vi "clipattconfiguration.vi"(0 "input cluster":T1, 1 "Channels values 2":i32[](array[numeric]), 2 "vclip":i32[](array[numeric]), 5 "Channels init":i32[](array[numeric])=[2000], 7 "Boolean":bool, 11 "error out 2":errorcluster) -> (6 "vatt":i32[](array[numeric]), 8 "vclip":i32[](array[numeric]), 10 "appended array":i64[](array[numeric]), 15 "error out":errorcluster)   [LabVIEW 2009]
uses:
  <vilib>/Utility/NIReport.llb/NI_report.lvclass
panel:
  in  "Array":dbl[](array[numeric])=[0.05, 0.1, 0.2, 0.3, 0.4, 0.5, 0.6, 0.7, 0.8, 0.9, 1.0, 1.2, 1.4, 1.6, 1.8, 2.0, 2.2, 2.5]
  in  "conf value":i32=100
  out "XY Graph":cluster{"Y":dbl[], "Y":dbl[]}[](graph)
  in  "L1 min invented 2":i32[](array[numeric])=[242, 504, 1031, 2128, 3263, 4418, 5634, 6888]
  in  "L1  50% invented 2":dbl[][](array[numeric])
  in  "L1  50% invented":dbl[][](array[numeric])
  in  "L1 min invented":i32[](array[numeric])=[242, 504, 1031, 2128, 3263, 4418, 5634, 6888]
  out "L1  50%":dbl[][](array[numeric])=[[182.05332645693656, 181.0458957661739, 182.31328051706822, 182.44384615384615, 179.9591580860661, 183.67138786049767, 183.0415079653926], [383.1443079334591, 380.3408546343534, 383.09068068207546, 382.9081242164992, 377.8888565224893, 386.4745006061593, 384.33733278296165], [789.794916143154, 783.9334435523022, 789.880331635444, 788.1638578058222, 779.1397265900023, 796.380113600458, 792.3805482207972], [1637.2849189817332, 1624.3008579976345, 1635.9791868307739, 1633.4037928039274, 1613.351662874732, 1647.9524154468106, 1640.5214046384517], [2513.43820756283, 2496.681867952526, 2512.120672224883, 2508.5174246445135, 2478.2432072662637, 2532.0838659445626, 2519.7319162836616], [4350.429616233692, 4325.797863663112, 4346.430175185175, 4343.835753463216, 4286.1263991243895, 4381.02010040906, 4360.577157137679], [5321.96395522116, 5291.780098348377, 5317.9835218197695, 5305.673007498198, 5228.362955923682, 5348.7398745375585, 5316.2612416656], [6878.716199794284, 6844.2297782699125, 6886.512941570447, 6849.728580417201, 6743.132495285984, 6910.301756503628, 6900.4988799604525]]
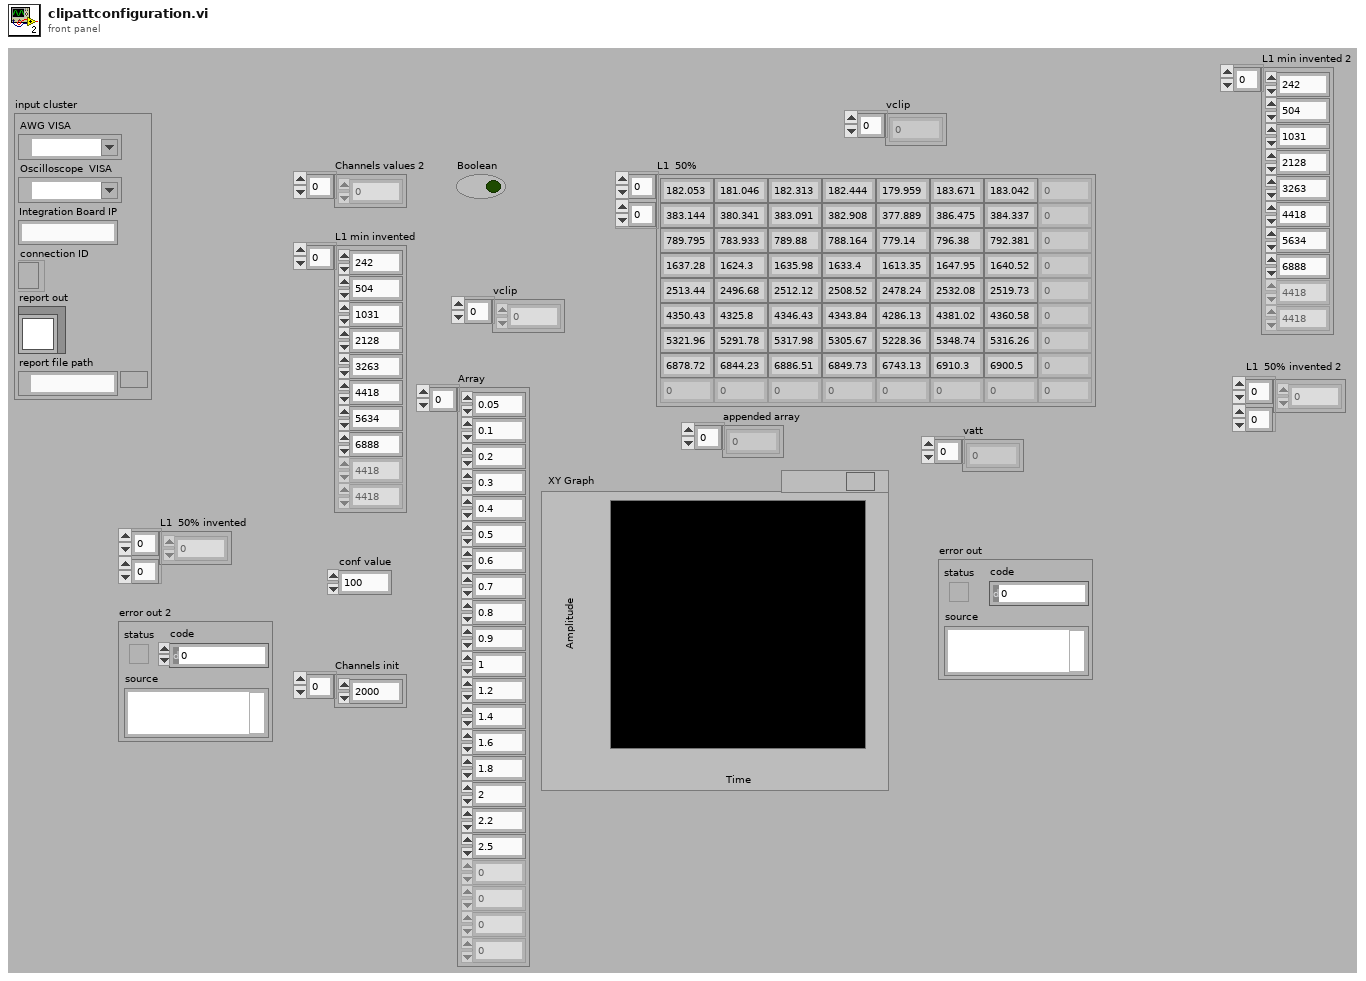
[diagram p1: front panel]
types:
  T1 = cluster{"AWG VISA":refnum<visa-resource-name>, "Oscilloscope  VISA ":refnum<visa-resource-name>, "Integration Board IP":string, "connection ID":refnum<k5>, "report out":refnum<class "NI_report.lvclass">, "report file path":path}
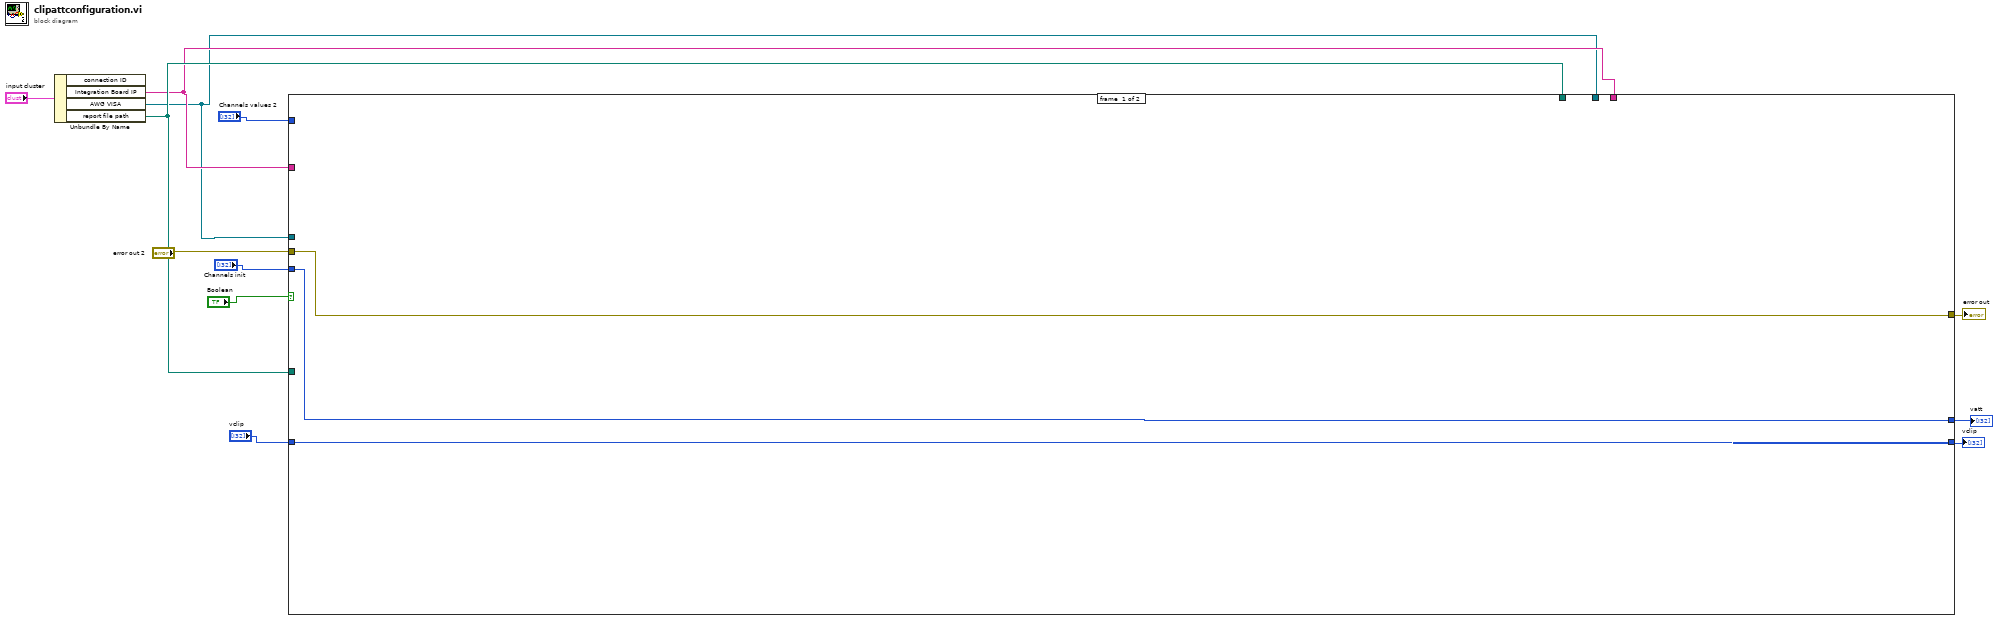
[diagram p0: block diagram]
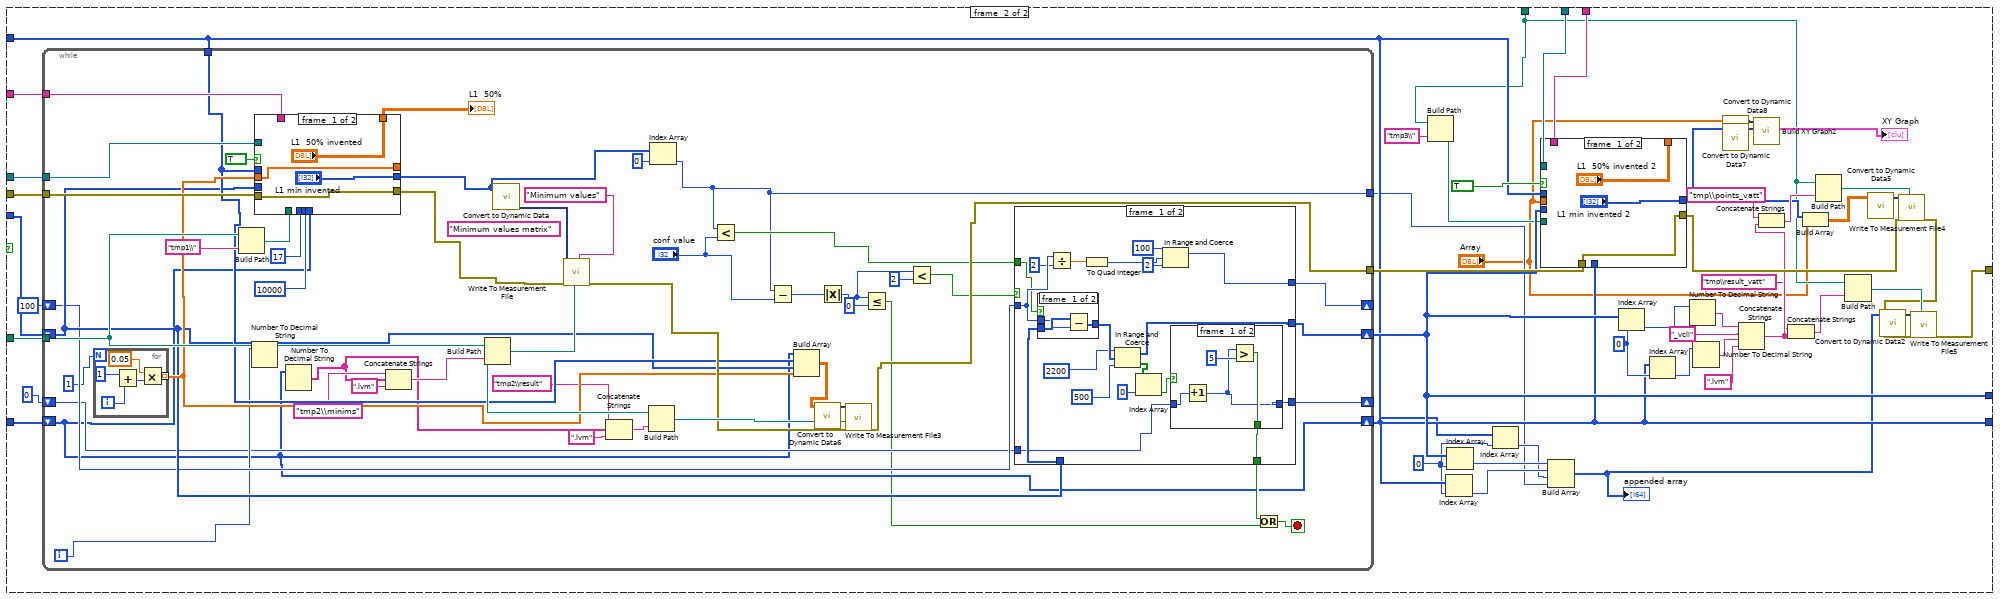
[diagram p2: hidden frame]
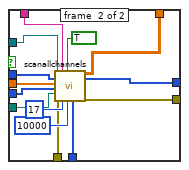
[diagram p3: hidden frame]
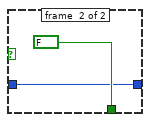
[diagram p4: hidden frame]
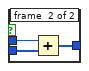
[diagram p5: hidden frame]
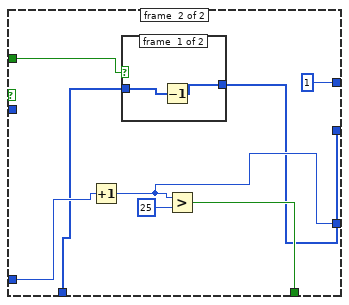
[diagram p6: hidden frame]
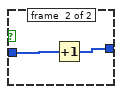
[diagram p7: hidden frame]
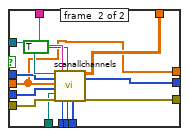
[diagram p8: hidden frame]
diagram:
  n1 = Unbundle By Name("input cluster") -> ("Integration Board IP"=w2:string, "AWG VISA"=w1:refnum<visa-resource-name>, "report file path"=w3:path)  [unwired: 1 out]
  n2 = case shown="True" "Boolean" {
    tunnel: "error out 2" -> [w15 w64]
    tunnel: w1 -> [_ w63]
    tunnel: w2 -> [_ w62]
    tunnel: w3 -> [_ w61]
    tunnel: [w13 w29] -> w8
    tunnel: "vclip" -> [w14 w60]
    tunnel: "Channels init" -> [w13 w59]
    tunnel: "Channels values 2" -> [_ w25]
    tunnel: [w15 w35] -> w12
    tunnel: [w14 w28] -> w4
    tunnel: w3 -> [_ w18]
    tunnel: w2 -> [_ w57]
    tunnel: w1 -> [_ w55]
    frame #0 {
    }
    frame #1 {
      w24 = 0 ("index")
      w51 = 0 ("index")
      n3 = while {
        tunnel: w64 -> [w128]
        tunnel: w63 -> [w127]
        tunnel: w62 -> [w126]
        tunnel: w61 -> [w121]
        tunnel: w25 -> [w115]
        tunnel: [w100] -> w56
        shift-right: [w105] -> w29
        shift-left: w59 -> [w106]
        shift-right: [w94] -> w28
        shift-left: w60 -> [w94]
        shift-right: [w104] -> _
        shift-left: 100 -> [w103]
        shift-right: [w98] -> _
        shift-left: 0 -> [w97]
        tunnel: [w82] -> w22
        i -> [w102]
        stop <- w96 stop-if-true
        (unwired) "Minimum values matrix" ("Comment")
        n4 = for {
          N: 1 -> [_]
          tunnel: [w175] -> w116 mode=indexing
          i -> [w179]
          n5 = Add(x=1, y=w179) -> (x+y=w177:i32)
          n6 = Multiply(x=0.05 ("y"), y=w177) -> (x*y=w175:dbl)
        }
        n7 = Build Path(base path=w121, name or relative path="tmp1\\") -> (appended path=w124:path)
        n8 = Number To Decimal String(number=w102) -> ()  [unwired: 1 in, 1 out]
        n9 = case shown="True" TRUE {
          tunnel: [w183 w197] -> w93
          tunnel: w128 -> [w183 w196]
          tunnel: w127 -> [_ w195]
          tunnel: w126 -> [_ w194]
          tunnel: w106 -> [_ w193]
          tunnel: w116 -> [w180 w184]
          tunnel: w115 -> [_ w192]
          tunnel: 17 ("Value") -> [_ w191]
          tunnel: 10000 ("Value") -> [_ w190]
          tunnel: ["L1 min invented" w188] -> w92
          tunnel: w124 -> [_ w187]
          tunnel: w94 -> [_ w186]
          tunnel: ["L1  50% invented" w185] -> w122
          tunnel: [w180 w184] -> _
          frame #0 {
          }
          frame #1 {
            n10 = call "scanallchannels.vi"("VISA resource name out"=w195, "nm ch"=w192, "Voltages values"=w184, "Init ch value"=w193, "base path"=w187, "error in"=w196, "Integration Board IP"=w194, "L1 Address"=w191, "Save test data"=TRUE, "Ch burst"=w190, "vclip"=w186) -> ("L1  50%"=w185:dbl[][], "L1 min values"=w188:i32[], "error out"=w197:errorcluster)  [unwired: 6 in]
          }
        }
        "L1  50%" <- w122
        n11 = Number To Decimal String(number=w94) -> (decimal integer string=w101:string[])  [unwired: 1 in]
        n12 = Concatenate Strings("tmp2\\minims" ("name or relative path"), w101, ".lvm" ("string")) -> (w112:string)
        n13 = Build Path(base path=w121, name or relative path=w112) -> (appended path=w129:path)
        n14 = call "Convert to Dynamic Data"("Array"=w92) -> ("Dynamic Data Type"=w131:dynamicdata)  [unwired: 3 in]
        n15 = call "Write To Measurement File"("Signals"=w131, "error in (no error)"=w93, "Filename"=w129, "Comment"="Minimum values") -> ("error out"=w119:errorcluster)  [unwired: 13 in, 2 out]
        n16 = Concatenate Strings("tmp2\\result" ("name or relative path"), w101, ".lvm" ("string")) -> (w109:string)
        n17 = Build Path(base path=w121, name or relative path=w109) -> (appended path=w120:path)
        n18 = Index Array(array=w92, index=0) -> (element=w82:i32)
        n19 = Less?(x=w82, y="conf value") -> (x < y?=w87:bool)
        n20 = Subtract(x=w82, y="conf value") -> (x-y=w88:i32)
        n21 = Build Array(w94, w115, w106, w116) -> (w118:dbl[][])
        n22 = call "Convert to Dynamic Data6"("2D Array"=w118) -> ("Dynamic Data Type"=w117:dynamicdata)  [unwired: 3 in]
        n23 = Absolute Value(x=w88) -> (abs(x)=w85:i32)
        n24 = call "Write To Measurement File3"("Signals"=w117, "error in (no error)"=w119, "Filename"=w120) -> ("error out"=w100:errorcluster)  [unwired: 14 in, 2 out]
        n25 = Less Or Equal?(x=w85, y=0) -> (x <= y?=w86:bool)
        n26 = Less?(x=w85, y=2) -> (x < y?=w83:bool)
        n27 = case shown="False" w83 {
          tunnel: w106 -> [w150 w166]
          tunnel: [w141 w165] -> w105
          tunnel: [w145 i64 1 ("upper limit")] -> w104
          tunnel: w103 -> [w149 _]
          tunnel: [w133 w167] -> w98
          tunnel: w97 -> [w134 w170]
          tunnel: [w132 w168] -> w95
          tunnel: w87 -> [w138 w163]
          frame #0 {
            n28 = case shown="True" w138 {
              tunnel: w150 -> [w159 w162]
              tunnel: w149 -> [w158 w161]
              tunnel: [w157 w160] -> w142
              frame #0 {
                n29 = Subtract(x=w159, y=w158) -> (x-y=w157:i64[])
              }
              frame #1 {
                n30 = Add(x=w161, y=w162) -> (x+y=w160:i64[])
              }
            }
            n31 = Divide(x=w149, y=2) -> (x/y=w147:dbl)
            n32 = To Quad Integer(1:w147) -> (0:w146:i64)
            n33 = In Range and Coerce(upper limit=i64 2200, x=w142, lower limit=i64 500 ("upper limit")) -> (coerced(x)=w141:i64[], In Range?=w137:bool[])
            n34 = Index Array(array=w137, index=0) -> (element=w135:bool)
            n35 = In Range and Coerce(upper limit=i64 100, x=w146, lower limit=i64 2) -> (coerced(x)=w145:i64)  [unwired: 1 out]
            n36 = case shown="False" w135 {
              tunnel: w134 -> [w152 w155]
              tunnel: [w151 w155] -> w133
              tunnel: [w153 FALSE] -> w132
              frame #0 {
                n37 = Increment(x=w152) -> (x+1=w151:i32)
                n38 = Greater?(x=w151, y=5) -> (0:w153:bool)
              }
              frame #1 {
              }
            }
          }
          frame #1 {
            n39 = Increment(x=w170) -> (x+1=w167:i32)
            n40 = case shown="True" w163 {
              tunnel: w166 -> [w171 w174]
              tunnel: [w172 w173] -> w165
              frame #0 {
                n41 = Decrement(x=w171) -> (x-1=w172:i64[])
              }
              frame #1 {
                n42 = Increment(x=w174) -> (x+1=w173:i64[])
              }
            }
            n43 = Greater?(x=w167, y=25) -> (0:w168:bool)
          }
        }
        n44 = Or(x=w95, y=w86) -> (x .or. y?=w96:bool)
      }
      n45 = Build Path(base path=w18, name or relative path="tmp3\\") -> (appended path=w17:path)
      n46 = Index Array(array=w28, index=w24) -> (element=w26:i32)
      n47 = Index Array(array=w29, index=w24) -> (element=w27:i64)
      n48 = Index Array(array=w25, index=w24) -> (element=w23:i32)
      n49 = case shown="True" TRUE {
        tunnel: [w65 w81] -> w52
        tunnel: ["L1 min invented 2" w79] -> w34
        tunnel: ["L1  50% invented 2" w78] -> _
        tunnel: "Array" -> [_ w77]
        tunnel: w28 -> [_ w74]
        tunnel: w29 -> [_ w73]
        tunnel: w17 -> [_ w72]
        tunnel: w57 -> [_ w71]
        tunnel: w56 -> [w65 w70]
        tunnel: w55 -> [_ w69]
        tunnel: w25 -> [_ w68]
        frame #0 {
        }
        frame #1 {
          n50 = call "scanallchannels.vi"("VISA resource name out"=w69, "nm ch"=w68, "Voltages values"=w77, "Init ch value"=w73, "base path"=w72, "error in"=w70, "Integration Board IP"=w71, "L1 Address"=17, "Save test data"=TRUE, "Ch burst"=10000, "vclip"=w74) -> ("L1  50%"=w78:dbl[][], "L1 min values"=w79:i32[], "error out"=w81:errorcluster)  [unwired: 6 in]
        }
      }
      n51 = Build Array(w27, w26, w23, w22) -> (w21:i64[])
      "appended array" <- w21
      n52 = Index Array(array=w29, index=w51) -> (element=w49:i64)
      n53 = Index Array(array=w28, index=w51) -> (element=w50:i32)
      n54 = Number To Decimal String(number=w49) -> (decimal integer string=w46:string)  [unwired: 1 in]
      n55 = Number To Decimal String(number=w50) -> (decimal integer string=w47:string)  [unwired: 1 in]
      n56 = call "Convert to Dynamic Data8"("Array"="Array") -> ("Dynamic Data Type"=w32:dynamicdata)  [unwired: 3 in]
      n57 = call "Convert to Dynamic Data7"("Array"=w34) -> ("Dynamic Data Type"=w33:dynamicdata)  [unwired: 3 in]
      n58 = Concatenate Strings(w46, "_vcli" ("string"), w47, ".lvm" ("string")) -> (w40:string)
      n59 = call "Build XY Graph2"("Y Input"=w33, "X Input"=w32) -> ("XY Graph"=→"XY Graph":cluster{"Y":dbl[], "Y":dbl[]}[])  [unwired: 8 in, 1 out]
      n60 = Concatenate Strings("tmp\\points_vatt" ("string"), w40) -> (w41:string)
      n61 = Concatenate Strings("tmp\\result_vatt" ("string"), w40) -> (w39:string)
      n62 = Build Array(w34, "Array") -> (w44:dbl[][])
      n63 = Build Path(base path=w18, name or relative path=w41) -> (appended path=w53:path)
      n64 = Build Path(base path=w18, name or relative path=w39) -> (appended path=w38:path)
      n65 = call "Convert to Dynamic Data5"("2D Array"=w44) -> ("Dynamic Data Type"=w43:dynamicdata)  [unwired: 3 in]
      n66 = call "Convert to Dynamic Data2"("Array"=w21) -> ("Dynamic Data Type"=w20:dynamicdata)  [unwired: 3 in]
      n67 = call "Write To Measurement File4"("Signals"=w43, "error in (no error)"=w52, "Filename"=w53) -> ("error out"=w36:errorcluster)  [unwired: 14 in, 2 out]
      n68 = call "Write To Measurement File5"("Signals"=w20, "error in (no error)"=w36, "Filename"=w38) -> ("error out"=w35:errorcluster)  [unwired: 14 in, 2 out]
    }
  }
  "error out" <- w12
  "vatt" <- w8
  "vclip" <- w4
